vi "Gamepad Tool.vi"() -> ()   [LabVIEW 2014]
doc: "Use this template to build a producer/consumer design pattern with events to produce queue items. Use this design pattern instead of the User Interface Event Handler pattern for user interfaces when you want to execute code asynchronously in response to an event without slowing the user interface responsiveness."
uses:
  <vilib>/Platform/browser.llb/Open URL in Default Browser (string).vi
panel:
  in  "Error":errorcluster
  in  "Info":bool
  out "Progress":u8(slide) scale=0.0..100.0
  in  "Program":bool
  in  "Scan":bool
  in  "Device":i32(listbox)=-1 caption="Select MSP430 Device"
  in  "Select Option":u16(ring) items=["Option 1", "Option 2", "Option 3"]
  out "MSP430 Pinout":picture
  # "Gamepad Tool For FRC"
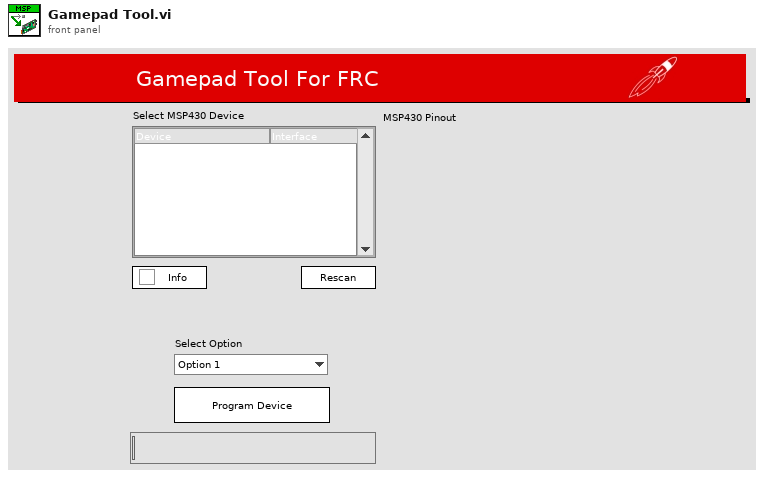
[diagram p1: front panel]
types:
  T1 = typedef "Config.ctl" = cluster{"Tool Path":path, "Firmware":path[], "Images":picture[], "Options":string[]}
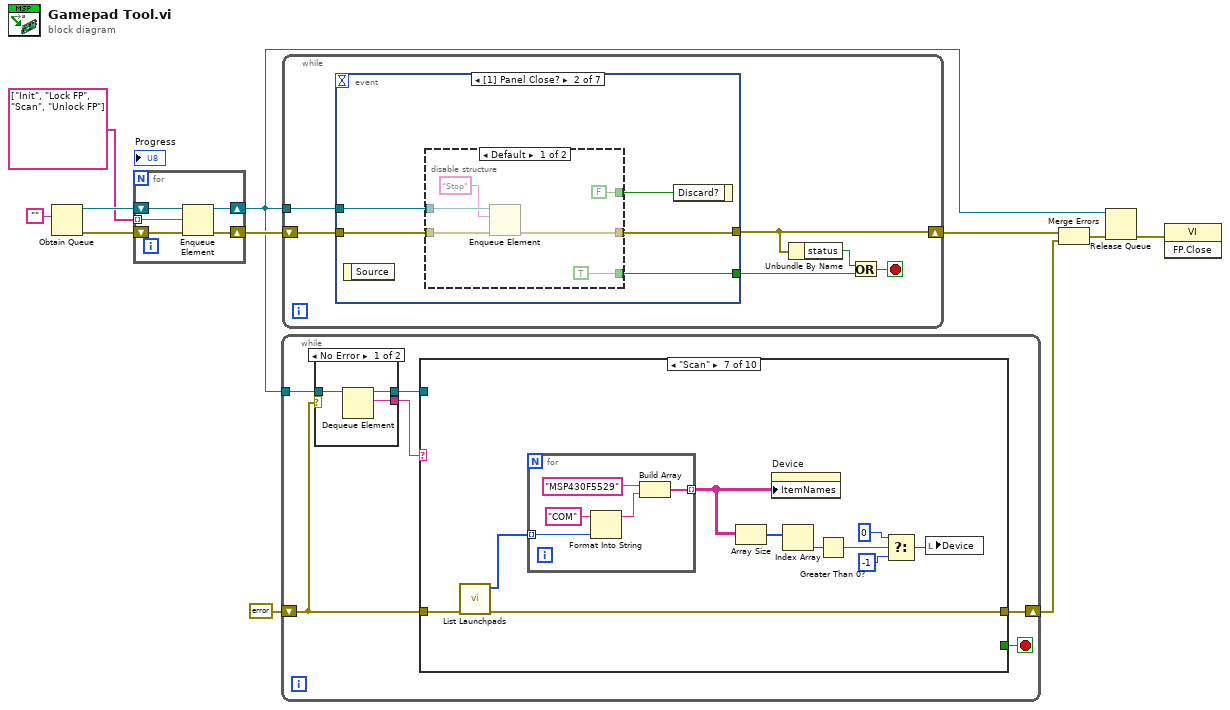
[diagram p0: block diagram]
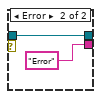
[diagram p2: hidden frame]
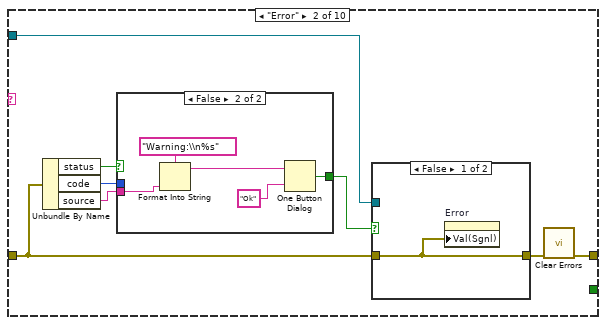
[diagram p4: hidden frame]
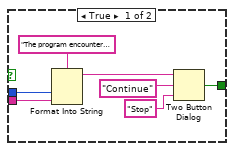
[diagram p5: hidden frame]
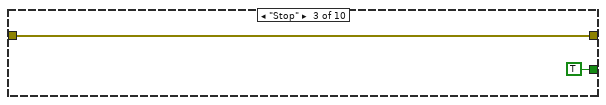
[diagram p7: hidden frame]
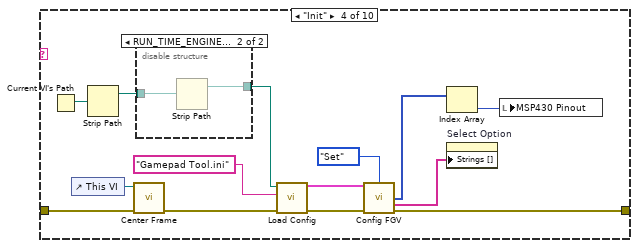
[diagram p8: hidden frame]
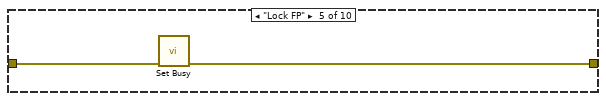
[diagram p10: hidden frame]
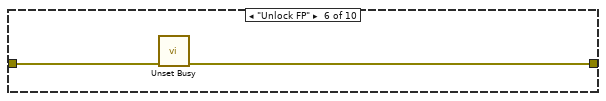
[diagram p11: hidden frame]
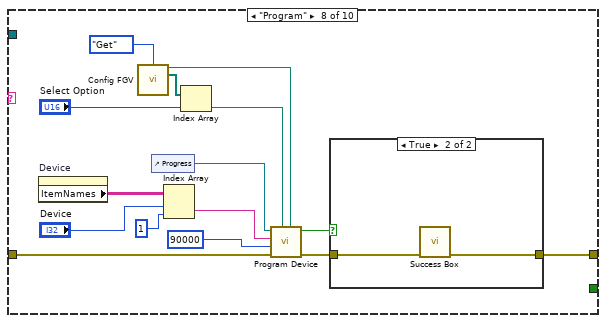
[diagram p12: hidden frame]
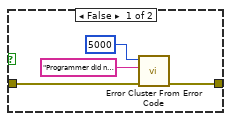
[diagram p13: hidden frame]
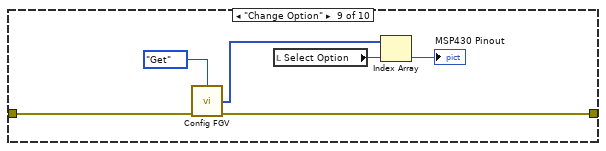
[diagram p14: hidden frame]
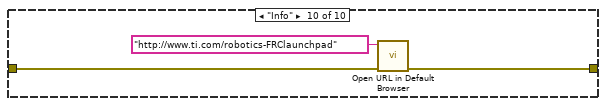
[diagram p15: hidden frame]
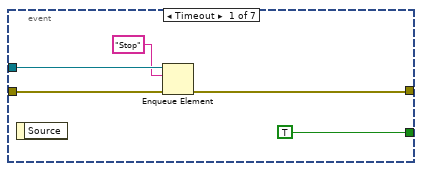
[diagram p16: hidden frame]
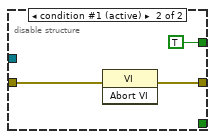
[diagram p17: hidden frame]
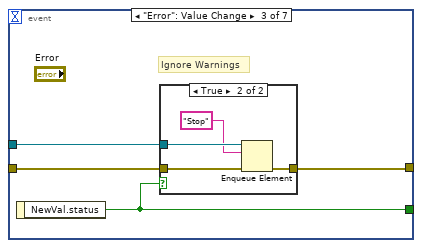
[diagram p18: hidden frame]
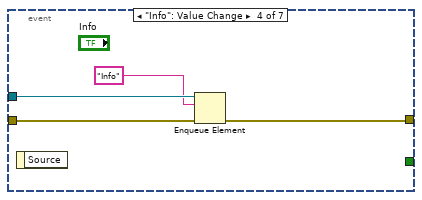
[diagram p20: hidden frame]
diagram:
  n1 = Obtain Queue(element data type="") -> (queue out=w8:refnum<queue>, error out=w11:errorcluster)  [unwired: 4 in, 1 out]
  n2 = for {
    shift-right: [w13] -> w7
    shift-left: w8 -> [w14]
    shift-right: [w15] -> w9
    shift-left: w11 -> [w16]
    tunnel: string[] ["Init", "Lock FP", "Scan", "Unlock FP"] -> [w12] mode=indexing
    n3 = Enqueue Element(queue=w14, element=w12, error in (no error)=w16) -> (queue out=w13:refnum<queue>, error out=w15:errorcluster)  [unwired: 1 in, 1 out]
  }
  n4 = while {
    tunnel: w7 -> [w22]
    shift-right: [w20] -> w5
    shift-left: errorcluster {"status"=FALSE, "code"=0, "source"=""} ("error out") -> [w17]
    stop <- w21 stop-if-true
    n5 = case shown="No Error" w17 {
      tunnel: w22 -> [w25 w27]
      tunnel: [w24 "Error"] -> w18
      tunnel: [w23 w27] -> w19
      frame No Error {
        n6 = Dequeue Element(queue=w25) -> (queue out=w23:refnum<queue>, element=w24:string)  [unwired: 2 in, 2 out]
      }
      frame Error {
      }
    }
    n7 = case shown="\"Scan\"" w18 {
      tunnel: [_ _ TRUE _ _ _ _ _ _ _] -> w21
      tunnel: [w28 w36 w51 w61 w71 w73 w82 w95 w114 w116] -> w20
      tunnel: w17 -> [w28 w32 w51 w65 w70 w72 w83 w103 w115 w118]
      tunnel: w19 -> [_ w30 _ _ _ _ _ _ _ _]
      frame Default {
      }
      frame "Error" {
        n8 = Unbundle By Name(w32) -> ("status"=w29:bool, "code"=w34:i32, "source"=w33:string)
        n9 = case shown="False" w29 {
          tunnel: w34 -> [w41 _]
          tunnel: w33 -> [w40 w45]
          tunnel: [w37 w44] -> w31
          frame True {
            n10 = Format Into String(format string="The program encountered an error: Error %d\\n%s", w41, w40) -> (resulting string=w38:string)  [unwired: 2 in, 1 out]
            n11 = Two Button Dialog(message=w38, 1:"Stop" ("F button name (\"Cancel\")"), 2:"Continue" ("T button name (\"OK\")")) -> (T button?=w37:bool)
          }
          frame False {
            n12 = Format Into String(format string="Warning:\\n%s", w45) -> (resulting string=w46:string)  [unwired: 2 in, 1 out]
            n13 = One Button Dialog(message=w46, button name ("OK")="Ok" ("T button name (\"OK\")")) -> (true=w44:bool)
          }
        }
        n14 = case shown="False" w31 {
          tunnel: [w49 w50] -> w35
          tunnel: w32 -> [w49 w50]
          tunnel: w30 -> [_ _]
          frame False {
            n15 = property on="Error" class="Clust (strict)"("Val(Sgnl)"=w49) -> ()  [unwired: 2 in, 2 out]
          }
          frame True {
          }
        }
        n16 = call <vilib>:"Clear Errors.vi"("error in (no error)"=w35) -> ("error out"=w36:errorcluster)  [unwired: 5 in, 1 out]
      }
      frame "Stop" {
      }
      frame "Init" {
        n17 = Current VI's Path() -> (path=w54:path)
        n18 = control-ref of="This VI"() -> (w66:refnum<vi>)
        n19 = Strip Path(path=w54) -> (stripped path=w53:path)  [unwired: 1 out]
        n20 = call "Center Frame.vi"("error in (no error)"=w65, "VI in"=w66) -> ("error out"=w64:errorcluster)  [unwired: 9 in]
        n21 = disable-structure shown="RUN_TIME_ENGINE==True" {
          disable-tunnel: [w67 w68] -> w55
          disable-tunnel: w53 -> [w67 w69]
          frame condition #0 (active) {
          }
          frame condition #1 {
            n22 = Strip Path(path=w69) -> (stripped path=w68:path)  [unwired: 1 out]
          }
        }
        n23 = call "Load Config.vi"("error in"=w64, "config"="Gamepad Tool.ini", "base path"=w55) -> ("error out"=w62:errorcluster, 3:w60:T1)  [unwired: 7 in]
        n24 = call "Config FGV.vi"("Data"=w60, "Operation"=enum16{"Get", "Set"}."Set", "error in"=w62) -> ("Images"=w57:picture[], "Options"=w59:string[], "error out"=w61:errorcluster)  [unwired: 8 in, 2 out]
        n25 = Index Array(array=w57) -> (element=w56:picture)  [unwired: 1 in]
        n26 = property on="Select Option" class="Ring (strict)"("Strings []"=w59) -> ()  [unwired: 2 in, 2 out]
        n27 = local write "MSP430 Pinout"(w56) -> ()
      }
      frame "Lock FP" {
        n28 = call <vilib>:"Set Busy.vi"("error in (no error)"=w70) -> ("error out"=w71:errorcluster)  [unwired: 9 in, 1 out]
      }
      frame "Unlock FP" {
        n29 = call <vilib>:"Unset Busy.vi"("error in (no error)"=w72) -> ("error out"=w73:errorcluster)  [unwired: 10 in]
      }
      frame "Scan" {
        n30 = call "List Launchpads.vi"("error in"=w83) -> ("error out"=w82:errorcluster, "Com Port"=w81:i32[])  [unwired: 8 in, 1 out]
        n31 = for {
          tunnel: w81 -> [w88] mode=indexing
          tunnel: [w84] -> w80 mode=indexing
          n32 = Format Into String(initial string="COM", w88) -> (resulting string=w85:string)  [unwired: 2 in, 1 out]
          n33 = Build Array("MSP430F5529" ("initial string"), w85) -> (w84:string[])
        }
        n34 = Array Size(array=w80) -> (size(s)=w79:i32[])
        n35 = property on="Device" class="MCListbox (strict)"("ItemNames"=w80) -> ()  [unwired: 2 in, 2 out]
        n36 = Index Array(array=w79) -> (element=w78:i32)  [unwired: 1 in]
        n37 = Greater Than 0?(x=w78) -> (x > 0?=w77:bool)
        n38 = Select(t=0, s=w77, f=-1) -> (s? t:f=w76:i32)
        n39 = local write "Device"(w76) -> ()
      }
      frame "Program" {
        n40 = property on="Device" class="MCListbox (strict)"() -> ("ItemNames"=w102:string[][])  [unwired: 2 in, 2 out]
        n41 = call "Config FGV.vi"("Operation"=enum16{"Get", "Set"}."Get") -> ("Tool Path"=w89:path, "Firmware"=w92:path[])  [unwired: 10 in, 3 out]
        n42 = control-ref of="Progress"() -> (w98:refnum<vi>)
        n43 = Index Array(array=w102, index (row)="Device", index (col)=1 ("disabled index (col)")) -> (element=w99:string)
        n44 = Index Array(array=w92, index="Select Option") -> (element=w91:path)
        n45 = call "Program Device.vi"("Tool Path"=w89, "Firmware Path"=w91, "error in"=w103, "Flash Timeout (ms)"=90000, "Com Port"=w99, "Slide in"=w98) -> ("error out"=w97:errorcluster, "Success"=w96:bool)  [unwired: 4 in]
        n46 = case shown="True" w96 {
          tunnel: w97 -> [w107 w109]
          tunnel: [w106 w108] -> w95
          frame False {
            n47 = call <vilib>:"Error Cluster From Error Code.vi"("error in (no error)"=w107, "error message (\"\")"="Programmer did not succeed. Check log for details" ("error message (\"\")"), "error code (0)"=5000) -> ("error out"=w106:errorcluster)  [unwired: 6 in]
          }
          frame True {
            n48 = call "Success Box.vi"("error in"=w109) -> ("error out"=w108:errorcluster)  [unwired: 10 in]
          }
        }
      }
      frame "Change Option" {
        n49 = call "Config FGV.vi"("Operation"=enum16{"Get", "Set"}."Get", "error in"=w115) -> ("Images"=w112:picture[], "error out"=w114:errorcluster)  [unwired: 9 in, 3 out]
        n50 = local read "Select Option"() -> (w111:u16)
        n51 = Index Array(array=w112, index=w111) -> (element=→"MSP430 Pinout":picture)
      }
      frame "Info" {
        n52 = call-poly <vilib>:"Open URL in Default Browser.vi"("error in (no error)"=w118, "URL"="http://www.ti.com/robotics-FRClaunchpad") -> ("error out"=w116:errorcluster)  [unwired: 4 in, 1 out]
      }
    }
  }
  n53 = while {
    shift-right: [w120] -> w6
    shift-left: w9 -> [w123]
    tunnel: w7 -> [w124]
    stop <- w121 stop-if-true
    n54 = event shown="[1] Panel Close?" {
      selector: _ -> [_ _ _ _ _ _ _]
      dyn-events: _ -> [_ _ _ _ _ _ _]
      timeout: _ -> [_ _ _ _ _ _ _]
      tunnel: w124 -> [w126 w132 w146 w155 w158 w166 w179]
      tunnel: w123 -> [w129 w134 w147 w156 w159 w167 w180]
      tunnel: [w127 w133 w145 w154 w160 w168 w181] -> w120
      tunnel: [TRUE ("stop") w131 w144 _ _ _ _] -> w122
      event Timeout {
        n55 = event-data() -> ()  [unwired: 1 in, 1 out]
        n56 = Enqueue Element(queue=w126, element="Stop", error in (no error)=w129) -> (error out=w127:errorcluster)  [unwired: 1 in, 2 out]
      }
      event Panel Close? {
        n57 = event-data() -> ()  [unwired: 1 in, 1 out]
        n58 = disable-structure shown="Default" {
          disable-tunnel: w134 -> [w140 w143]
          disable-tunnel: [w139 w142] -> w133
          disable-tunnel: w132 -> [w138 _]
          disable-tunnel: [TRUE ("stop") _] -> w131
          disable-tunnel: [FALSE TRUE] -> w130
          frame condition #0 {
            n59 = Enqueue Element(queue=w138, element="Stop", error in (no error)=w140) -> (error out=w139:errorcluster)  [unwired: 1 in, 2 out]
          }
          frame condition #1 (active) {
            n60 = invoke class="VI" method="Abort VI"(error in=w143) -> (error out=w142:errorcluster)  [unwired: 2 in, 2 out]
          }
        }
        n61 = event-data("Discard?"=w130) -> ()  [unwired: 1 in, 1 out]
      }
      event "Error": Value Change {
        # "Ignore Warnings"
        n62 = event-data() -> ("NewVal.status"=w144:bool)  [unwired: 1 in]
        n63 = case shown="True" w144 {
          tunnel: w147 -> [w148 w152]
          tunnel: w146 -> [_ w151]
          tunnel: [w148 w149] -> w145
          frame False {
          }
          frame True {
            n64 = Enqueue Element(queue=w151, element="Stop", error in (no error)=w152) -> (error out=w149:errorcluster)  [unwired: 1 in, 2 out]
          }
        }
      }
      event "Info": Value Change {
        n65 = event-data() -> ()  [unwired: 1 in, 1 out]
        n66 = Enqueue Element(queue=w155, element="Info", error in (no error)=w156) -> (error out=w154:errorcluster)  [unwired: 1 in, 2 out]
      }
      event "Scan": Value Change {
        n67 = event-data() -> ()  [unwired: 1 in, 1 out]
        n68 = for {
          tunnel: w158 -> [w162]
          shift-right: [w164] -> w160
          shift-left: w159 -> [w163]
          tunnel: string[] ["Lock FP", "Scan", "Unlock FP"] -> [w161] mode=indexing
          n69 = Enqueue Element(queue=w162, element=w161, error in (no error)=w163) -> (error out=w164:errorcluster)  [unwired: 1 in, 2 out]
        }
      }
      event "Program": Value Change {
        n70 = event-data() -> ()  [unwired: 1 in, 1 out]
        n71 = local read "Device"() -> (w165:i32)
        n72 = case shown="0, Default" w165 {
          tunnel: [w169 w173] -> w168
          tunnel: w167 -> [w169 w172]
          tunnel: w166 -> [_ w171]
          frame -1 {
          }
          frame 0, Default {
            n73 = for {
              tunnel: w171 -> [w175]
              shift-right: [w177] -> w173
              shift-left: w172 -> [w176]
              tunnel: string[] ["Lock FP", "Program", "Unlock FP"] -> [w174] mode=indexing
              n74 = Enqueue Element(queue=w175, element=w174, error in (no error)=w176) -> (error out=w177:errorcluster)  [unwired: 1 in, 2 out]
            }
          }
        }
      }
      event "Select Option": Value Change {
        n75 = event-data() -> ()  [unwired: 1 in, 1 out]
        n76 = for {
          tunnel: w179 -> [w183]
          shift-right: [w185] -> w181
          shift-left: w180 -> [w184]
          tunnel: string[] ["Change Option"] -> [w182] mode=indexing
          n77 = Enqueue Element(queue=w183, element=w182, error in (no error)=w184) -> (error out=w185:errorcluster)  [unwired: 1 in, 2 out]
        }
      }
    }
    n78 = Unbundle By Name(w120) -> ("status"=w119:bool)
    n79 = Or(x=w119, y=w122) -> (x .or. y?=w121:bool)
  }
  n80 = Merge Errors(w6, w5) -> (w4:errorcluster)
  n81 = Release Queue(queue=w7, error in (no error)=w4) -> (error out=w1:errorcluster)  [unwired: 1 in, 2 out]
  n82 = invoke class="VI" method="FP.Close"(error in=w1) -> ()  [unwired: 2 in, 3 out]
